vi "GetAllBufferedNephData.vi"(7 "LabVIEW Web Service Request":refnum<class "Web Request.lvclass">, 10 "Format":string caption="Format (use accept header)", 11 "Measurement":string caption="Measurement (all)") -> ()   [LabVIEW 2013]
uses:
  <vilib>/wsapi/Web Request.lvclass
  Nephelometer/NephDataEnum.ctl
  Nephelometer/NephDataCluster.ctl
  C:/Program Files (x86)/National Instruments/LabVIEW 2013/examples/Connectivity/Web Services/Weather Monitor/Application/Weather Data.lvlib
panel:
  # "Use the Web Service Request input terminal to call the VIs on the Web Services palette. Do not remove it from the connector pane unless you don't need access to the palette."
  # "Each additional control wired to the connector pane will be available as an input in the URL. To include an indicator in terminal-mode output (the default setting), it must also be wired to the connector pane."
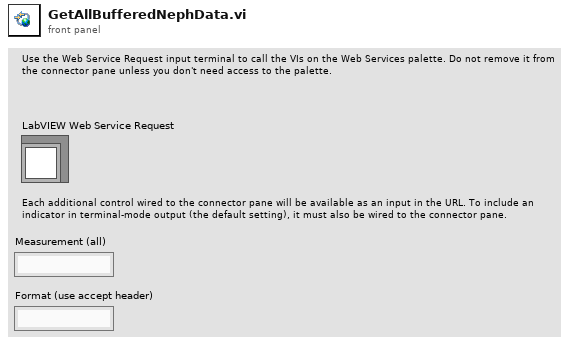
[diagram p1: front panel]
types:
  T1 = typedef "NephDataCluster.ctl" = cluster{"dateTime":string, "unitNo":string, "RF_PMT":dbl, "RF_REF":dbl, "GF_PMT":dbl, "GF_REF":dbl, "BF_PMT":dbl, "BF_REF":dbl, "RB_PMT":dbl, "RB_REF":dbl, "GB_PMT":dbl, "GB_REF":dbl, "BB_PMT":dbl, "BB_REF":dbl, "Temp":dbl, "Pressure":dbl, "RH":dbl, "PMT_DARK":dbl, "Forw_Dark_Ref":dbl, "Back_Dark_Ref":dbl, "Back_Scatt_Red":dbl, "Back_Scatt_Green":dbl, "Back_Scatt_Blue":dbl, "Total_Scatt_Red":dbl, "Total_Scatt_Green":dbl, "Total_Scatt_Blue":dbl, "Fan_RPM":dbl}
  T2 = typedef "NephDataEnum.ctl" = enum16{"Init", "Insert Measurement", "Read Buffer Size", "Write Buffer Size", "Read Current Measurement", "Read All Buffered Meas"}
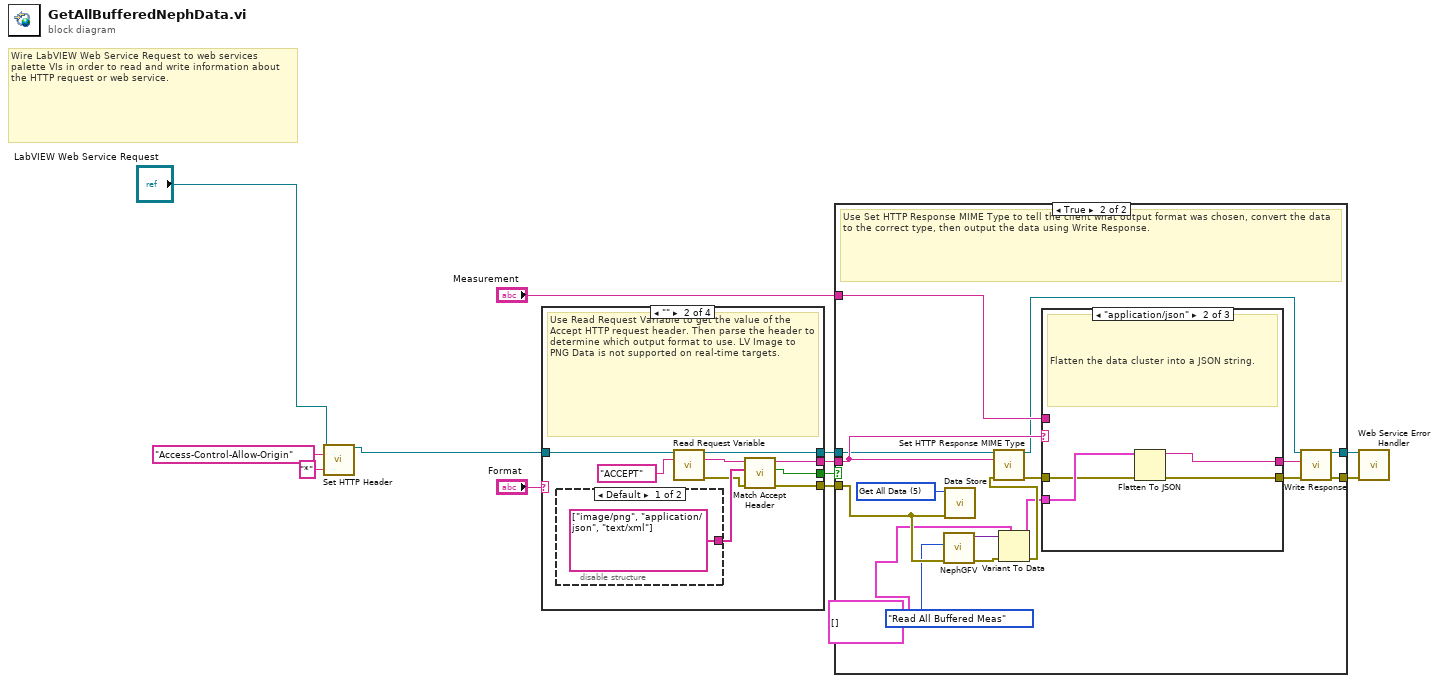
[diagram p0: block diagram]
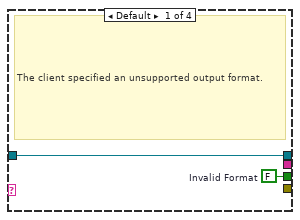
[diagram p2: hidden frame]
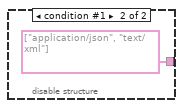
[diagram p3: hidden frame]
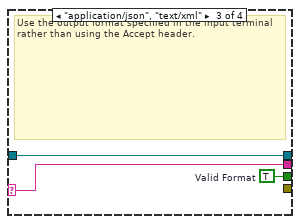
[diagram p4: hidden frame]
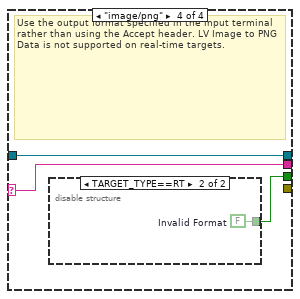
[diagram p5: hidden frame]
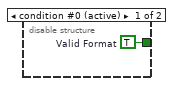
[diagram p6: hidden frame]
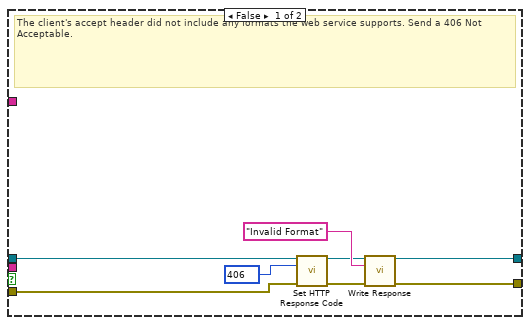
[diagram p7: hidden frame]
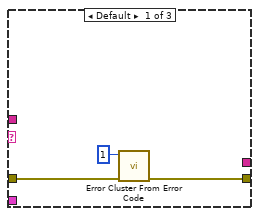
[diagram p8: hidden frame]
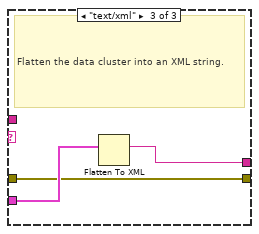
[diagram p9: hidden frame]
diagram:
  # "Wire LabVIEW Web Service Request to web services palette VIs in order to read and write information about the HTTP request or web service."
  n1 = call <vilib>:"Set HTTP Header.vi"("LabVIEW Web Service Request"="LabVIEW Web Service Request", "header"="Access-Control-Allow-Origin", "header value"="*") -> ("LabVIEW Web Service Request out"=w4:refnum<class "Web Request.lvclass">)  [unwired: 11 in, 1 out]
  n2 = case shown="\"\"" "Format" {
    selector: "Format" -> [_ _ w27 w30]
    tunnel: w4 -> [w14 w15 w28 w31]
    tunnel: [w13 w20 w26 w29] -> w12
    tunnel: [w14 w19 w28 w31] -> w11
    tunnel: [_ w17 _ _] -> w10
    tunnel: [_ w16 w27 w30] -> w9
    frame Default {
      w13 = FALSE  # Invalid Format
      # "The client specified an unsupported output format."
    }
    frame "" {
      # "Use Read Request Variable to get the value of the Accept HTTP request header. Then parse the header to determine which output format to use. LV Image to PNG Data is not supported on real-time targets."
      n3 = disable-structure shown="Default" {
        disable-tunnel: [string[] ["image/png", "application/json", "text/xml"] ("Valid Media Types") string[] ["application/json", "text/xml"] ("Valid Media Types")] -> w21
        frame condition #0 (active) {
        }
        frame condition #1 {
        }
      }
      n4 = call <vilib>:"Read Request Variable.vi"("LabVIEW Web Service Request"=w15, "variable name"="ACCEPT") -> ("LabVIEW Web Service Request out"=w19:refnum<class "Web Request.lvclass">, "value"=w22:string, "error out"=w18:errorcluster)  [unwired: 11 in]
      n5 = call "Match Accept Header.vi"("error in (no error)"=w18, "Valid Media Types"=w21, "Accept Value"=w22) -> ("error out"=w17:errorcluster, "Matched?"=w20:bool, "Matched Media Type"=w16:string)  [unwired: 6 in]
    }
    frame "application/json", "text/xml" {
      w26 = TRUE  # Valid Format
      # "Use the output format specified in the input terminal rather than using the Accept header."
    }
    frame "image/png" {
      # "Use the output format specified in the input terminal rather than using the Accept header. LV Image to PNG Data is not supported on real-time targets."
      n6 = disable-structure shown="TARGET_TYPE==RT" {
        disable-tunnel: [w32 w33] -> w29
        frame condition #0 (active) {
          w32 = TRUE  # Valid Format
        }
        frame condition #1 {
          w33 = FALSE  # Invalid Format
        }
      }
    }
  }
  n7 = case shown="True" w12 {
    tunnel: w11 -> [w35 w50]
    tunnel: w10 -> [w40 w48]
    tunnel: w9 -> [_ w57]
    tunnel: "Measurement" -> [_ w51]
    tunnel: [w37 w53] -> w7
    tunnel: [w36 w52] -> w6
    frame False {
      w41 = 406 items=["100"=100, "101"=101, "200"=200, "201"=201, "202"=202, "203"=203, "204"=204, "205"=205, "206"=206, "300"=300, "301"=301, "302"=302, "303"=303, "304"=304, "305"=305, "306"=306, "307"=307, "400"=400, "401"=401, "402"=402, "403"=403, "404"=404, "405"=405, "406"=406, "407"=407, "408"=408, "409"=409, "410"=410, "411"=411, "412"=412, "413"=413, "414"=414, "415"=415, "416"=416, "417"=417, "500"=500, "501"=501, "502"=502, "503"=503, "504"=504, "505"=505] ("response code (200)")
      # "The client's accept header did not include any formats the web service supports. Send a 406 Not Acceptable."
      n8 = call <vilib>:"Set HTTP Response Code.vi"("LabVIEW Web Service Request"=w35, "response code (200)"=w41, "error in (no error)"=w40) -> ("LabVIEW Web Service Request out"=w34:refnum<class "Web Request.lvclass">, "error out"=w39:errorcluster)  [unwired: 11 in]
      n9 = call <vilib>:"Write Response.vi"("LabVIEW Web Service Request"=w34, "response string"="Invalid Format", "error in (no error)"=w39) -> ("LabVIEW Web Service Request out"=w36:refnum<class "Web Request.lvclass">, "error out"=w37:errorcluster)  [unwired: 11 in]
    }
    frame True {
      w56 = u16 5 items=["Initialize Data Store", "Destroy Data Store", "Clear Data", "Append Data", "Get Last Data", "Get All Data"] ("action")
      # "Use Set HTTP Response MIME Type to tell the client what output format was chosen, convert the data to the correct type, then output the data using Write Response."
      n10 = call "NephGFV.vi"("error in (no error)"=w48, "NephDataEnum"=NephDataEnum."Read All Buffered Meas") -> ("error out"=w46:errorcluster, "Variant Out"=w43:variant)  [unwired: 8 in]
      n11 = call "Data Store.vi"("error in (no error)"=w48, "action"=w56) -> ()  [unwired: 8 in, 2 out]
      n12 = Variant To Data(error in=w46, type=T1[] [] ("initialized array"), Variant=w43) -> (data=w44:T1[], error out=w45:errorcluster)
      n13 = call <vilib>:"Set HTTP Response MIME Type.vi"("LabVIEW Web Service Request"=w50, "MIME type (text/html)"=w57, "error in (no error)"=w45) -> ("LabVIEW Web Service Request out"=w49:refnum<class "Web Request.lvclass">, "error out"=w58:errorcluster)  [unwired: 11 in]
      n14 = case shown="\"application/json\"" w57 {
        tunnel: w58 -> [w61 w64 w67]
        tunnel: w44 -> [_ w65 w68]
        tunnel: [w60 w62 w67] -> w54
        tunnel: [_ w63 w66] -> w55
        tunnel: w51 -> [_ _ _]
        frame Default {
          n15 = call <vilib>:"Error Cluster From Error Code.vi"("error in (no error)"=w61, "error code (0)"=1) -> ("error out"=w60:errorcluster)  [unwired: 7 in]
        }
        frame "application/json" {
          # "Flatten the data cluster into a JSON string."
          n16 = Flatten To JSON(anything=w65, error in (no error)=w64) -> (JSON string=w63:string, 11:w62:errorcluster)  [unwired: 1 in]
        }
        frame "text/xml" {
          # "Flatten the data cluster into an XML string."
          n17 = Flatten To XML(anything=w68) -> (xml string=w66:string)
        }
      }
      n18 = call <vilib>:"Write Response.vi"("LabVIEW Web Service Request"=w49, "response string"=w55, "error in (no error)"=w54) -> ("LabVIEW Web Service Request out"=w52:refnum<class "Web Request.lvclass">, "error out"=w53:errorcluster)  [unwired: 11 in]
    }
  }
  n19 = call "Web Service Error Handler.vi"("LabVIEW Web Service Request"=w6, "error in (no error)"=w7) -> ()  [unwired: 12 in, 2 out]
